vi "Register Dynamic Events.vi"(8 "error in (no error)":errorcluster, 11 "VIEventHandler In":refnum<class "VIEventHandler.lvclass">) -> (0 "error out":errorcluster, 3 "VIEventHandler Out":refnum<class "VIEventHandler.lvclass">)   [LabVIEW 2020, in "ActorEvents.lvlib" / "VIEventHandler.lvclass"]
uses:
  <vilib>/gpm_packages/@cs/mva-viewable/Source/ActorEvents/EventHandler/VIEventHandler/VIEventHandler.lvclass
  C:/Program Files/National Instruments/LabVIEW 2020/vi.lib/gpm_packages/@cs/mva-viewable/Source/ActorEvents/IEventHandler/IEventHandler.lvclass
  <vilib>/gpm_packages/@cs/mva-viewable/Source/ActorEvents/IEventHandler/IEventHandler.lvclass/IEventHandler.ctl
  <vilib>/event_ctls.llb/lveventtype.ctl
  <vilib>/gpm_packages/@cs/mva-viewable/Source/ActorEvents/EventHandler/VIEventHandler/VIEventHandler.lvclass/VIEventHandler.ctl
  <vilib>/gpm_packages/@cs/mva-viewable/Source/ActorEvents/IEventHandler/Read Registrations.vi
  <vilib>/gpm_packages/@cs/mva-viewable/Source/ActorEvents/IEventHandler/IEventHandler.lvclass
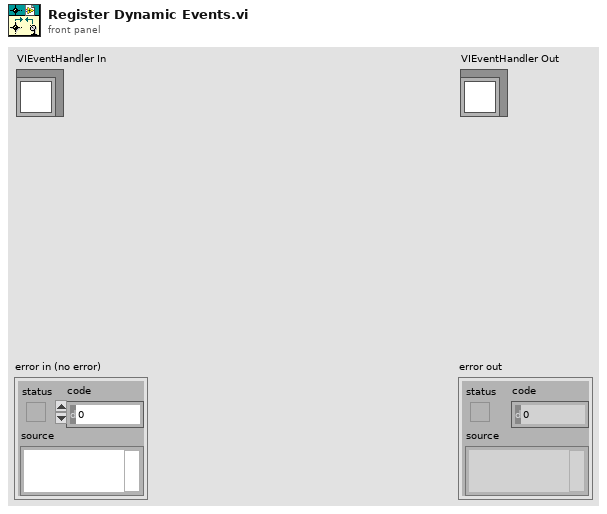
[diagram p1: front panel]
types:
  T1 = typedef "lveventtype.ctl" = enum32{"Null", "Timeout", "Annotation Menu Selection", "Annotation Menu Selection?", "App Instance Close", "App Instance Close?", "Autoscale Range Change", "Bookmark Info Change", "Cell Edit", "Cell Edit?", "Cursor Grab", "Cursor Grab?", "Cursor Menu Selection", "Cursor Menu Selection?", "Cursor Move", "Cursor Release", "Data Change", "Direction Change", "Display State Change", "Drag Ended", "Drag Enter", "Drag Leave", "Drag Over", "Drag Source Update", "Drag Starting", "Drag Starting?", "Drop", "Exec State Change", "Key Down", "Key Down?", "Key Repeat", "Key Repeat?", "Key Up", "Listbox Double Click", "Menu Activation?", "Menu Selection (App)", "Menu Selection? (App)", "Menu Selection (User)", "Mouse Down", "Mouse Down?", "Mouse Enter", "Mouse Leave", "Mouse Move", "Mouse Up", "Mouse Wheel", "NI Security User Change (App)", "Pane Size", "Panel Close", "Panel Close?", "Panel Resize", "Plot Attribute Change", "Scale Range Change", "Shortcut Menu Activation?", "Shortcut Menu Selection (App)", "Shortcut Menu Selection? (App)", "Shortcut Menu Selection (User)", "Tree Double Click", "Tree Drag", "Tree Drag?", "Tree Drop", "Tree Drop?", "Tree Item Close", "Tree Item Close?", "Tree Item Open", "Tree Item Open?", "User Event", "Value Change"}
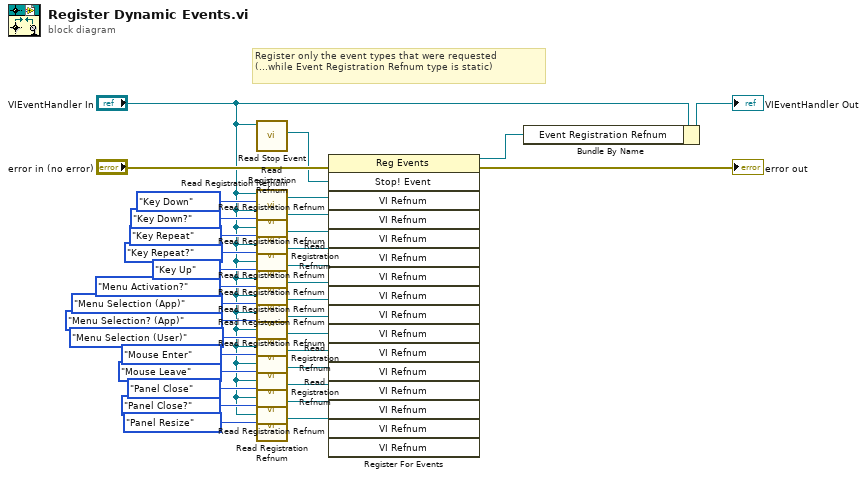
[diagram p0: block diagram]
diagram:
  # "Register only the event types that were requested\n(...while Event Registration Refnum type is static)"
  n1 = call <vilib>:"Read Stop Event.vi"("IEventHandler in"="VIEventHandler In") -> ("Stop! Event"=w31:refnum<user-event>)  [unwired: 10 in]
  n2 = call <vilib>:"Read Registration Refnum.vi"("Event Type"=lveventtype."Key Down", "VIEventHandler"="VIEventHandler In") -> ("VI Refnum"=w30:refnum<vi>)  [unwired: 5 in]
  n3 = call <vilib>:"Read Registration Refnum.vi"("Event Type"=lveventtype."Key Down?", "VIEventHandler"="VIEventHandler In") -> ("VI Refnum"=w28:refnum<vi>)  [unwired: 5 in]
  n4 = call <vilib>:"Read Registration Refnum.vi"("Event Type"=lveventtype."Key Repeat", "VIEventHandler"="VIEventHandler In") -> ("VI Refnum"=w27:refnum<vi>)  [unwired: 5 in]
  n5 = call <vilib>:"Read Registration Refnum.vi"("Event Type"=lveventtype."Key Repeat?", "VIEventHandler"="VIEventHandler In") -> ("VI Refnum"=w26:refnum<vi>)  [unwired: 5 in]
  n6 = call <vilib>:"Read Registration Refnum.vi"("Event Type"=lveventtype."Key Up", "VIEventHandler"="VIEventHandler In") -> ("VI Refnum"=w25:refnum<vi>)  [unwired: 5 in]
  n7 = call <vilib>:"Read Registration Refnum.vi"("Event Type"=lveventtype."Menu Activation?", "VIEventHandler"="VIEventHandler In") -> ("VI Refnum"=w24:refnum<vi>)  [unwired: 5 in]
  n8 = call <vilib>:"Read Registration Refnum.vi"("Event Type"=lveventtype."Menu Selection (App)", "VIEventHandler"="VIEventHandler In") -> ("VI Refnum"=w23:refnum<vi>)  [unwired: 5 in]
  n9 = call <vilib>:"Read Registration Refnum.vi"("Event Type"=lveventtype."Menu Selection? (App)", "VIEventHandler"="VIEventHandler In") -> ("VI Refnum"=w22:refnum<vi>)  [unwired: 5 in]
  n10 = call <vilib>:"Read Registration Refnum.vi"("Event Type"=lveventtype."Menu Selection (User)", "VIEventHandler"="VIEventHandler In") -> ("VI Refnum"=w21:refnum<vi>)  [unwired: 5 in]
  n11 = call <vilib>:"Read Registration Refnum.vi"("Event Type"=lveventtype."Mouse Enter", "VIEventHandler"="VIEventHandler In") -> ("VI Refnum"=w20:refnum<vi>)  [unwired: 5 in]
  n12 = call <vilib>:"Read Registration Refnum.vi"("Event Type"=lveventtype."Mouse Leave", "VIEventHandler"="VIEventHandler In") -> ("VI Refnum"=w19:refnum<vi>)  [unwired: 5 in]
  n13 = call <vilib>:"Read Registration Refnum.vi"("Event Type"=lveventtype."Panel Close", "VIEventHandler"="VIEventHandler In") -> ("VI Refnum"=w18:refnum<vi>)  [unwired: 5 in]
  n14 = call <vilib>:"Read Registration Refnum.vi"("Event Type"=lveventtype."Panel Close?", "VIEventHandler"="VIEventHandler In") -> ("VI Refnum"=w17:refnum<vi>)  [unwired: 5 in]
  n15 = call <vilib>:"Read Registration Refnum.vi"("Event Type"=lveventtype."Panel Resize", "VIEventHandler"="VIEventHandler In") -> ("VI Refnum"=w29:refnum<vi>)  [unwired: 5 in]
  n16 = register-events(error in="error in (no error)", w31, w30, w28, w27, w26, w25, w24, w23, w22, w21, w20, w19, w18, w17, w29) -> (reference out=w2:refnum<event-registration>, error out=→"error out":errorcluster)  [unwired: 1 in]
  n17 = Bundle By Name(cluster="VIEventHandler In", "Event Registration Refnum"=w2) -> (→"VIEventHandler Out":refnum<class "VIEventHandler.lvclass">)
